vi "Cleanup.vi"(8 "error in (no error)":errorcluster, 11 "CReporter in":refnum<class "CReporter.lvclass">) -> (0 "error out":errorcluster, 3 "CReporter out":refnum<class "CReporter.lvclass">)   [LabVIEW 2020, in "DependencyInspection.lvlib" / "CReporter.lvclass"]
uses:
  CReporter.lvclass
  CDependencyList/CDependencyList.lvclass
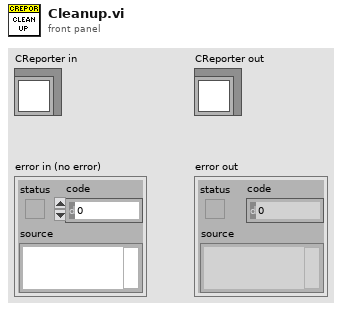
[diagram p1: front panel]
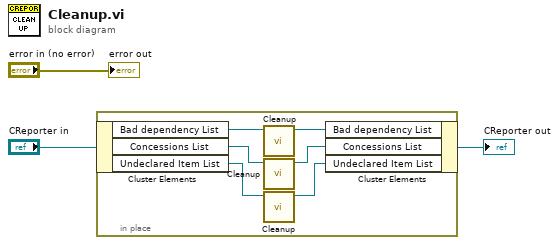
[diagram p0: block diagram]
diagram:
  n1 = in-place {
    n2 = in-place-cluster #1("CReporter in") -> ("Bad dependency List"=w9:refnum<class "CDependencyList.lvclass">, "Concessions List"=w7:refnum<class "CDependencyList.lvclass">, "Undeclared Item List"=w6:refnum<class "CDependencyList.lvclass">)
    n3 = call-dynamic "Cleanup.vi"("CDependencyList in"=w9) -> ("CDependencyList out"=w8:refnum<class "CDependencyList.lvclass">)  [unwired: 9 in, 1 out]
    n4 = call-dynamic "Cleanup.vi"("CDependencyList in"=w7) -> ("CDependencyList out"=w5:refnum<class "CDependencyList.lvclass">)  [unwired: 9 in, 1 out]
    n5 = call-dynamic "Cleanup.vi"("CDependencyList in"=w6) -> ("CDependencyList out"=w4:refnum<class "CDependencyList.lvclass">)  [unwired: 9 in, 1 out]
    n6 = in-place-cluster #1("Bad dependency List"=w8, "Concessions List"=w5, "Undeclared Item List"=w4) -> (→"CReporter out":refnum<class "CReporter.lvclass">)
  }
  "error out" <- "error in (no error)"
